vi "Replace BD Constant.vi"(8 "error in (no error)":errorcluster, 11 "Setter Generator In":refnum<class "API VI Generator.lvclass">) -> (0 "error out":errorcluster, 3 "Setter Generator Out":refnum<class "API VI Generator.lvclass">)   [LabVIEW 2020, in "Method Generation.lvlib" / "API VI Generator.lvclass"]
uses:
  API VI Generator.lvclass
  <vilib>/Utility/traverseref.llb/TRef TravTarget.ctl
  API VI Generator.lvclass/API VI Generator.ctl
  <vilib>/Utility/traverseref.llb/VI Scripting - Traverse.lvlib
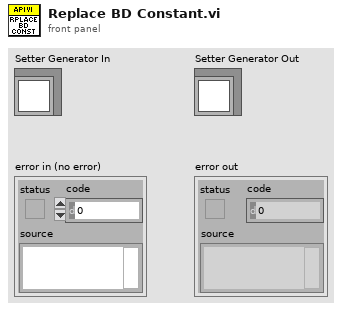
[diagram p1: front panel]
types:
  T1 = typedef "TRef TravTarget.ctl" = enum16{"FP", "BD", "Other"}
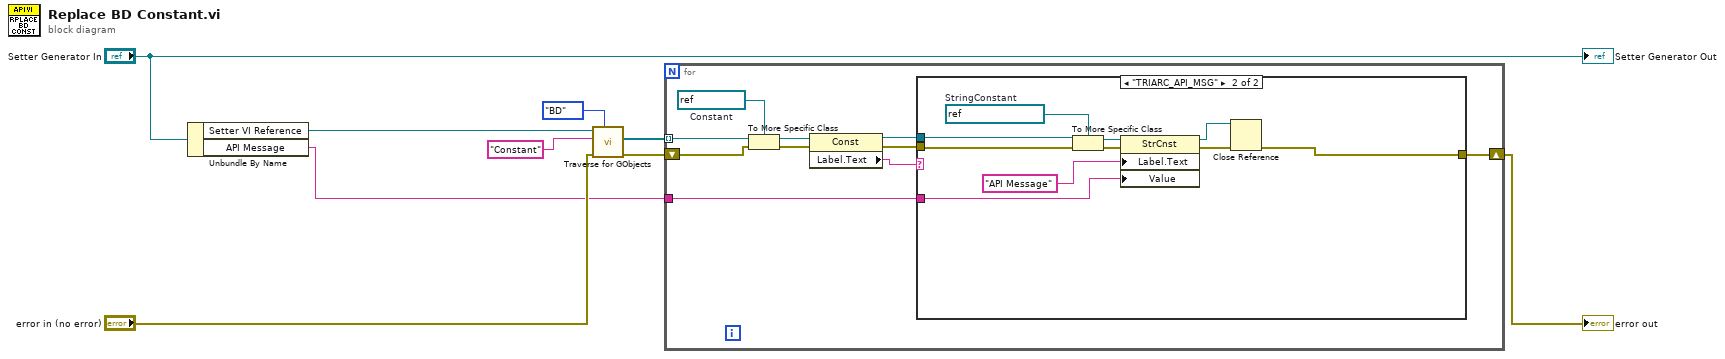
[diagram p0: block diagram]
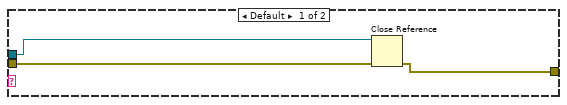
[diagram p2: hidden frame]
diagram:
  n1 = Unbundle By Name("Setter Generator In") -> ("Setter VI Reference"=w5:refnum<vi>, "API Message"=w1:string)
  n2 = call <vilib>:"Traverse for GObjects.vi"("Traverse Target"=TRef_TravTarget."BD", "error in (no error)"="error in (no error)", "Class Name"="Constant", "VI Refnum"=w5) -> ("error out"=w3:errorcluster, "References"=w4:refnum<vi>[])  [unwired: 4 in, 2 out]
  n3 = for {
    tunnel: w4 -> [w19] mode=indexing
    shift-right: [w17] -> w2
    shift-left: w3 -> [w18]
    tunnel: w1 -> [w10]
    w16 = refnum<vi> refnum  # Constant
    n4 = To More Specific Class(target class=w16, reference=w19, error in=w18) -> (specific class reference=w13:refnum<vi>, error out=w15:errorcluster)
    n5 = property class="Const"(reference=w13, error in=w15) -> (reference out=w12:refnum<vi>, error out=w14:errorcluster, "Label.Text"=w11:string)
    n6 = case shown="\"TRIARC_API_MSG\"" w11 {
      tunnel: [w21 w26] -> w17
      tunnel: w14 -> [w22 w31]
      tunnel: w12 -> [w20 w32]
      tunnel: w10 -> [_ w23]
      frame Default {
        n7 = Close Reference(reference=w20, error in (no error)=w22) -> (error out=w21:errorcluster)
      }
      frame "TRIARC_API_MSG" {
        w30 = refnum<vi> refnum  # StringConstant
        n8 = To More Specific Class(target class=w30, reference=w32, error in=w31) -> (specific class reference=w29:refnum<vi>, error out=w28:errorcluster)
        n9 = property class="StrCnst"(reference=w29, error in=w28, "Label.Text"="API Message", "Value"=w23) -> (reference out=w25:refnum<vi>, error out=w27:errorcluster)
        n10 = Close Reference(reference=w25, error in (no error)=w27) -> (error out=w26:errorcluster)
      }
    }
  }
  "error out" <- w2
  "Setter Generator Out" <- "Setter Generator In"
